vi "close methods.vi"(8 "error in (no error)":errorcluster, 11 "Method Manager in":refnum<class "Method Loader.lvclass">) -> (0 "error out":errorcluster)   [LabVIEW 2017, in "Method Loader.lvclass"]
uses:
  Method Loader.lvclass
  method type.ctl
  Method Loader.lvclass/Method Loader.ctl
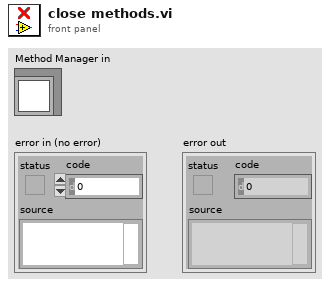
[diagram p1: front panel]
types:
  T1 = typedef "Method Loader.lvclass/method type.ctl" = refnum<vi>
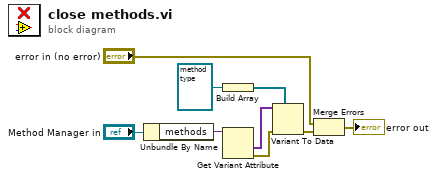
[diagram p0: block diagram]
diagram:
  n1 = Unbundle By Name("Method Manager in") -> ("methods"=w1:variant)
  n2 = Build Array(T1 refnum ("type specifier VI Refnum (for type only)")) -> (w7:T1[])
  n3 = Get Variant Attribute(Variant=w1) -> (values=w5:variant[], error out=w8:errorcluster)  [unwired: 3 in, 2 out]
  n4 = Variant To Data(error in=w8, type=w7, Variant=w5) -> (error out=w3:errorcluster)  [unwired: 1 out]
  n5 = Merge Errors("error in (no error)", w3) -> (→"error out":errorcluster)
